vi "_gStop.vi"(6 "op":enum16{"reset", "get", "stop"}(ring)=enum."stop", 8 "error in (no error)":errorcluster) -> (0 "error out":errorcluster, 3 "Boolean":bool)   [LabVIEW 2013, in "GlobalStop(dev).lvlib"]
uses:
  GlobalStop(dev).lvlib
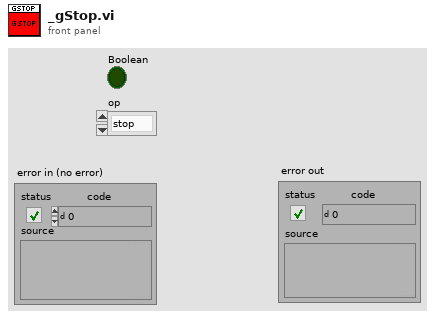
[diagram p1: front panel]
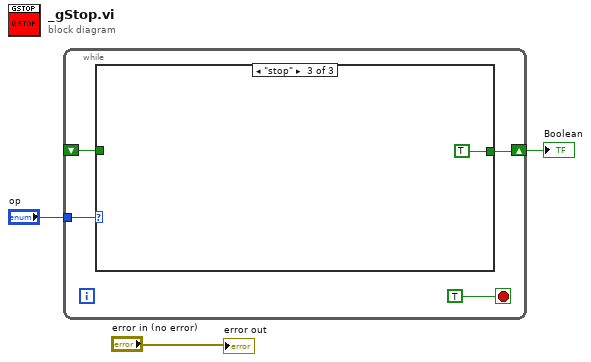
[diagram p0: block diagram]
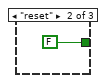
[diagram p3: hidden frame]
diagram:
  n1 = while {
    tunnel: "op" -> [w6]
    shift-right: [w5] -> w2
    shift-left: _ -> [w4]
    stop <- TRUE stop-if-true
    n2 = case shown="\"stop\"" w6 {
      tunnel: [w8 FALSE TRUE] -> w5
      tunnel: w4 -> [w8 _ _]
      frame "get", Default {
      }
      frame "reset" {
      }
      frame "stop" {
      }
    }
  }
  "Boolean" <- w2
  "error out" <- "error in (no error)"
